vi "SetValve.vi"(8 "error in":errorcluster, 10 "ON":bool=TRUE, 11 "Valve":u16=999) -> (0 "error out":errorcluster)   [LabVIEW 2013]
uses:
  GlobalVariables/ValveValues.vi
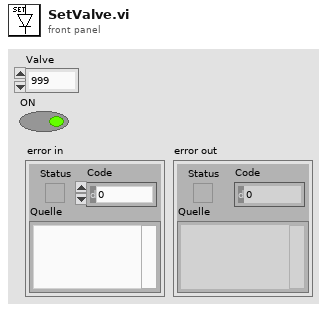
[diagram p1: front panel]
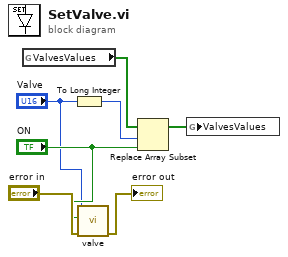
[diagram p0: block diagram]
diagram:
  n1 = global read "ValveValues.vi" "ValvesValues"() -> (w5:bool[])
  n2 = To Long Integer(number="Valve") -> (32bit integer=w7:i32)
  n3 = call "valve.vi"("error in"="error in", "ON"="ON", "Valve"="Valve") -> ("error out"=→"error out":errorcluster)  [unwired: 8 in]
  n4 = Replace Array Subset(array=w5, new element="ON", index=w7) -> (w6:bool[])
  n5 = global write "ValveValues.vi" "ValvesValues"(w6) -> ()
